vi "evaluate_expression.vi"(8 "error in (no error)":errorcluster, 9 "images in":refnum<class "Image.lvclass">[](array[class]), 10 "term in":string, 11 "destination image in":refnum<class "Image.lvclass">) -> (0 "error out":errorcluster, 3 "result out":refnum<class "Image.lvclass">)   [LabVIEW 2010, in "Image.lvclass"]
uses:
  Image.lvclass
  ErrorController/ErrorController/class_data.vi
  ErrorController/ErrorController/ErrorController.lvclass
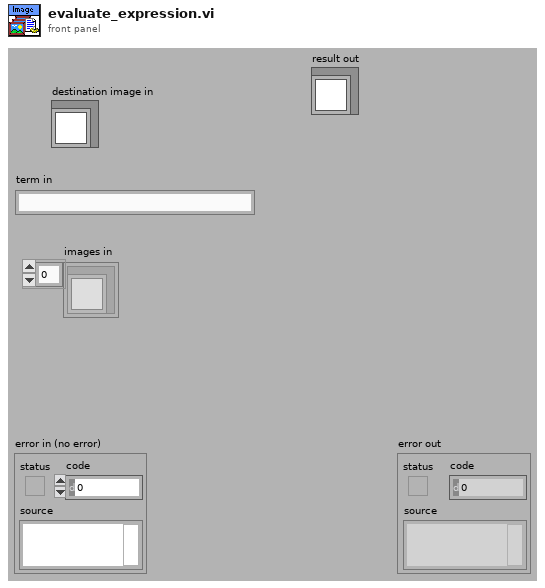
[diagram p1: front panel]
types:
  T1 = typedef "Image Type" = u32
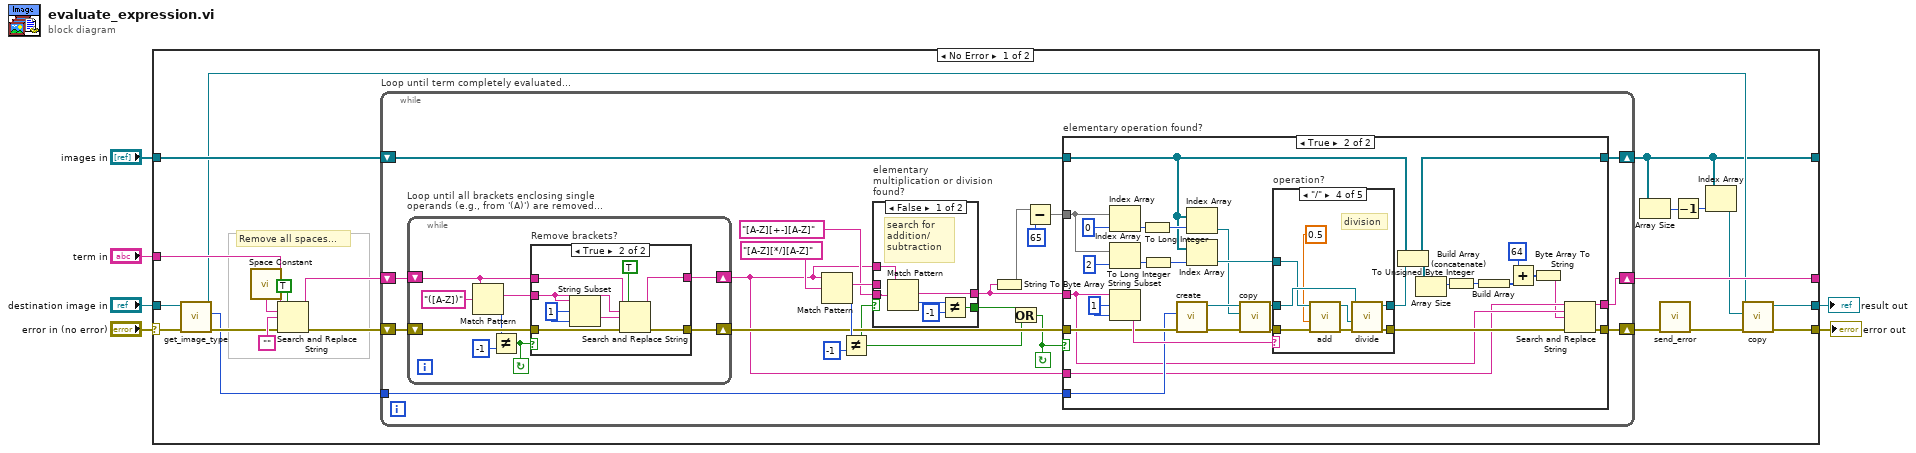
[diagram p0: block diagram]
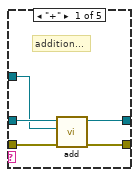
[diagram p4: hidden frame]
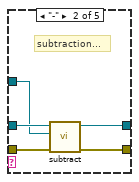
[diagram p5: hidden frame]
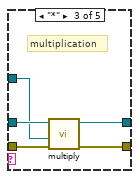
[diagram p6: hidden frame]
diagram:
  n1 = case shown="No Error" "error in (no error)" {
    selector: "error in (no error)" -> [w20 w136]
    tunnel: [w15 w136] -> w5
    tunnel: "term in" -> [w27 _]
    tunnel: "images in" -> [w21 w135]
    tunnel: [w12 w135] -> _
    tunnel: [w16 _] -> _
    tunnel: "destination image in" -> [w18 w134]
    tunnel: [w13 w134] -> w1
    frame No Error {
      # "Remove all spaces..."
      n2 = call-dynamic "get_image_type.vi"("error in (no error)"=w20, "Image.lvclass in"=w18) -> ("error out"=w19:errorcluster, "Image Type"=w17:T1, "Image.lvclass out"=w14:refnum<class "Image.lvclass">)  [unwired: 7 out]
      n3 = call <vilib>:"Space Constant.vi"() -> ("String"=w26:string)
      n4 = Search and Replace String(replace all?=TRUE ("replace all? (F)"), input string=w27, search string=w26, replace string="", error in=w19) -> (result string=w22:string, error out=w23:errorcluster)  [unwired: 5 out]
      n5 = while "Loop until term completely evaluated..." {
        tunnel: w17 -> [w36]
        shift-right: [w40] -> w12
        shift-left: w21 -> [w41]
        shift-right: [w42] -> w8
        shift-left: w23 -> [w47]
        shift-right: [w35] -> w16
        shift-left: w22 -> [w46]
        stop <- w28 continue-if-true
        n6 = while "Loop until all brackets enclosing single operands (e.g., from '(A)') are removed..." {
          shift-right: [w121] -> w43
          shift-left: w47 -> [w122]
          shift-right: [w120] -> w31
          shift-left: w46 -> [w115]
          stop <- w116 continue-if-true
          n7 = Match Pattern(string=w115, regular expression="([A-Z])") -> (match substring=w119:string, offset past match=w118:i32)  [unwired: 3 out]
          n8 = Not Equal?(x=w118, y=-1) -> (x != y?=w116:bool)
          n9 = case "Remove brackets?" shown="True" w116 {
            tunnel: w122 -> [w124 w133]
            tunnel: [w124 w132] -> w121
            tunnel: w115 -> [w125 w130]
            tunnel: [w125 w129] -> w120
            tunnel: w119 -> [_ w127]
            frame False {
            }
            frame True {
              w128 = 1 ("offset (0)")
              n10 = String Subset(string=w127, offset (0)=w128, length (rest)=w128) -> (substring=w126:string)
              n11 = Search and Replace String(replace all?=TRUE ("replace all? (F)"), input string=w130, search string=w127, replace string=w126, error in=w133) -> (result string=w129:string, error out=w132:errorcluster)  [unwired: 5 out]
            }
          }
        }
        n12 = Match Pattern(string=w31, regular expression="[A-Z][*/][A-Z]") -> (match substring=w34:string, offset past match=w44:i32)  [unwired: 3 out]
        n13 = Not Equal?(x=w44, y=-1) -> (x != y?=w29:bool)
        n14 = case "elementary multiplication or division found?" shown="False" w29 {
          tunnel: w34 -> [_ w55]
          tunnel: [w54 w55] -> w33
          tunnel: "[A-Z][+-][A-Z]" ("regular expression") -> [w53 _]
          tunnel: w31 -> [w52 _]
          tunnel: [w49 _] -> w30
          frame False {
            # "search for addition/subtraction"
            n15 = Match Pattern(string=w52, regular expression=w53) -> (match substring=w54:string, offset past match=w50:i32)  [unwired: 3 out]
            n16 = Not Equal?(x=w50, y=-1) -> (x != y?=w49:bool)
          }
          frame True {
          }
        }
        n17 = String To Byte Array(string=w33) -> (unsigned byte array=w39:u8[])
        n18 = Or(x=w30, y=w29) -> (x .or. y?=w28:bool)
        n19 = Subtract(x=w39, y=u8 65) -> (x-y=w38:u8[])
        n20 = case "elementary operation found?" shown="True" w28 {
          tunnel: w43 -> [w58 w79]
          tunnel: [w58 w69] -> w42
          tunnel: w41 -> [w57 w71]
          tunnel: [w57 w65] -> w40
          tunnel: w38 -> [_ w88]
          tunnel: w33 -> [_ w68]
          tunnel: w36 -> [_ w78]
          tunnel: w31 -> [w56 w67]
          tunnel: [w56 w66] -> w35
          frame False {
          }
          frame True {
            w86 = 1 ("offset (0)")
            n21 = Index Array(array=w88, index=0 ("offset (0)")) -> (element=w84:u8)
            n22 = Index Array(array=w88, index=2 ("offset (0)")) -> (element=w82:u8)
            n23 = String Subset(string=w68, offset (0)=w86, length (rest)=w86) -> (substring=w85:string)
            n24 = To Long Integer(number=w84) -> (32bit integer=w83:i32)
            n25 = To Long Integer(number=w82) -> (32bit integer=w81:i32)
            n26 = call "create.vi"("error in (no error)"=w79, "Image Type"=w78) -> ("error out"=w77:errorcluster, "Image out"=w75:refnum<class "Image.lvclass">)  [unwired: 2 in, 6 out]
            n27 = Index Array(array=w71, index=w83) -> (element=w74:refnum<class "Image.lvclass">)
            n28 = Index Array(array=w71, index=w81) -> (element=w80:refnum<class "Image.lvclass">)
            n29 = call "copy.vi"("error in (no error)"=w77, "image to copy (source)"=w74, "Image in (target)"=w75) -> ("error out"=w76:errorcluster, "Image out"=w73:refnum<class "Image.lvclass">)  [unwired: 7 out]
            n30 = case "operation?" shown="\"/\"" w85 {
              tunnel: w76 -> [w92 w99 w104 w110 w114]
              tunnel: [w91 w98 w103 w112 w114] -> w70
              tunnel: w80 -> [w90 w95 w101 w106 _]
              tunnel: w73 -> [w94 w97 w102 w107 w113]
              tunnel: [w93 w96 w100 w111 w113] -> w72
              frame "+" {
                # "addition..."
                n31 = call-dynamic "add.vi"("error in (no error)"=w92, "addend"=w90, "Image in"=w94) -> ("error out"=w91:errorcluster, "Image out"=w93:refnum<class "Image.lvclass">)  [unwired: 1 in, 6 out]
              }
              frame "-" {
                # "subtraction..."
                n32 = call-dynamic "subtract.vi"("error in (no error)"=w99, "subtrahend"=w95, "Image in"=w97) -> ("error out"=w98:errorcluster, "Image out"=w96:refnum<class "Image.lvclass">)  [unwired: 7 out]
              }
              frame "*" {
                # "multiplication"
                n33 = call-dynamic "multiply.vi"("error in (no error)"=w104, "factor image"=w101, "Image in"=w102) -> ("error out"=w103:errorcluster, "Image out"=w100:refnum<class "Image.lvclass">)  [unwired: 1 in, 6 out]
              }
              frame "/" {
                # "division"
                n34 = call-dynamic "add.vi"("error in (no error)"=w110, "constant"=sgl 0.5, "Image in"=w106) -> ("error out"=w109:errorcluster, "Image out"=w108:refnum<class "Image.lvclass">)  [unwired: 1 in, 6 out]
                n35 = call-dynamic "divide.vi"("error in (no error)"=w109, "divisor"=w108, "Image in"=w107) -> ("error out"=w112:errorcluster, "Image out"=w111:refnum<class "Image.lvclass">)  [unwired: 1 in, 6 out]
              }
              frame Default {
                # "none (should not happen anyway)..."
              }
            }
            n36 = Build Array (concatenate)(w71, w72) -> (w65:refnum<class "Image.lvclass">[])
            n37 = Array Size(array=w65) -> (size(s)=w64:i32)
            n38 = To Unsigned Byte Integer(number=w64) -> (unsigned 8bit integer=w63:u8)
            n39 = Build Array(w63) -> (w61:u8[])
            n40 = Add(x=u8 64, y=w61) -> (x+y=w60:u8[])
            n41 = Byte Array To String(unsigned byte array=w60) -> (string=w59:string)
            n42 = Search and Replace String(input string=w67, search string=w68, replace string=w59, error in=w70) -> (result string=w66:string, error out=w69:errorcluster)  [unwired: 6 out]
          }
        }
      }
      n43 = Array Size(array=w12) -> (size(s)=w10:i32)
      n44 = call "send_error.vi"("error in (no error)"=w8) -> ("error out"=w7:errorcluster)  [unwired: 10 in]
      n45 = Decrement(x=w10) -> (x-1=w11:i32)
      n46 = Index Array(array=w12, index=w11) -> (element=w9:refnum<class "Image.lvclass">)
      n47 = call "copy.vi"("error in (no error)"=w7, "image to copy (source)"=w9, "Image in (target)"=w14) -> ("error out"=w15:errorcluster, "Image out"=w13:refnum<class "Image.lvclass">)  [unwired: 7 out]
    }
    frame Error {
    }
  }
  "error out" <- w5
  "result out" <- w1
